vi "Build_Igus_CanOpen.vi"(7 "Read (F) / Write":bool, 8 "error in (no error)":errorcluster, 9 "Data [1-4]":u8[](array[numeric]) format="%.0x", 10 "Sub Index":u8 format="%.0x", 11 "Address":u16 format="%.0x") -> (0 "error out":errorcluster, 3 "MB_PDU":T1={"Function Code"=1, "Data"=[], "RTU_DataBytes"=0})   [LabVIEW 2016, in "MB Master.lvlib"]
doc: "Builds PDU for Read Device Identification (function code 43 / 14)."
uses:
  MB Master.lvlib
  MB_PDU_Cluster.ctl
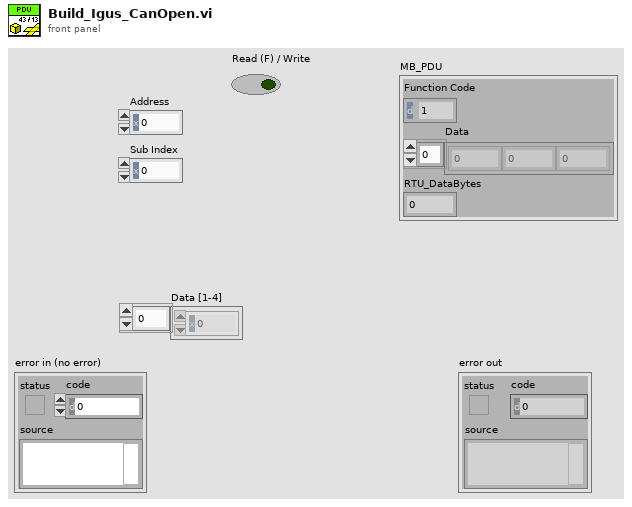
[diagram p1: front panel]
types:
  T1 = typedef "MB Master.lvlib/MB_PDU_Cluster.ctl" = cluster{"Function Code":u8, "Data":u8[], "RTU_DataBytes":i32}
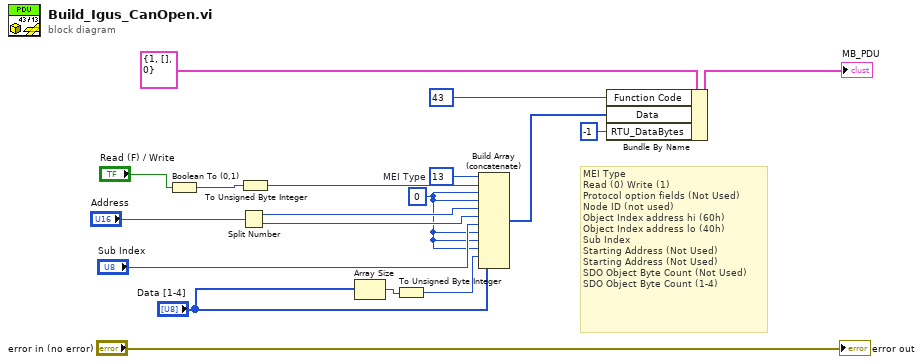
[diagram p0: block diagram]
diagram:
  w5 = u8 0
  w12 = u8 13  # MEI Type
  # "MEI Type\nRead (0) Write (1)\nProtocol option fields (Not Used)\nNode ID (not used)\nObject Index address hi (60h)\nObject Index address lo (40h)\nSub Index\nStarting Address (Not Used)\nStarting Address (Not Used)\nSDO Object Byte Count (Not Used)\nSDO Object Byte Count (1-4)"
  n1 = Boolean To (0,1)(Boolean="Read (F) / Write") -> (0, 1=w2:i16)
  n2 = Split Number(x="Address") -> (hi(x)=w9:u8, lo(x)=w8:u8)
  n3 = To Unsigned Byte Integer(number=w2) -> (unsigned 8bit integer=w1:u8)
  n4 = Array Size(array="Data [1-4]") -> (size(s)=w6:i32)
  n5 = To Unsigned Byte Integer(number=w6) -> (unsigned 8bit integer=w4:u8)
  n6 = Build Array (concatenate)(w12, w1, w5, w5, w9, w8, "Sub Index", w5, w5, w5, w4, "Data [1-4]") -> (w14:u8[])
  n7 = Bundle By Name(cluster=T1 {"Function Code"=1, "Data"=[], "RTU_DataBytes"=0} ("Modbus Serial New.lvlib:MB_PDU.lvclass"), "Function Code"=u8 43, "Data"=w14, "RTU_DataBytes"=-1) -> (→"MB_PDU":T1)
  "error out" <- "error in (no error)"
